vi "Change Color.vi"(8 "error in (no error)":errorcluster, 10 "Color Box":u32, 11 "GObject in":refnum<vi>) -> (0 "error out":errorcluster)   [LabVIEW 2013]
uses:
  Controls/Security System Indicators.ctl
panel:
  out "Zone status indicators":T1
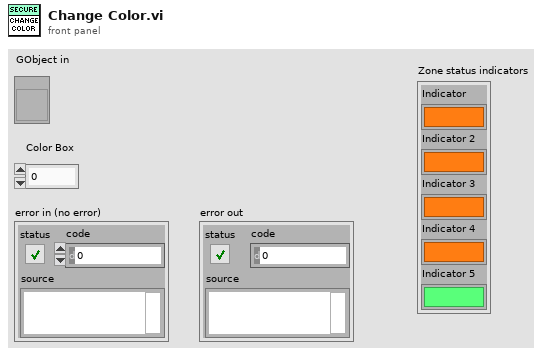
[diagram p1: front panel]
types:
  T1 = typedef "Security System Indicators.ctl" = cluster{"Indicator":bool, "Indicator 2":bool, "Indicator 3":bool, "Indicator 4":bool, "Indicator 5":bool}
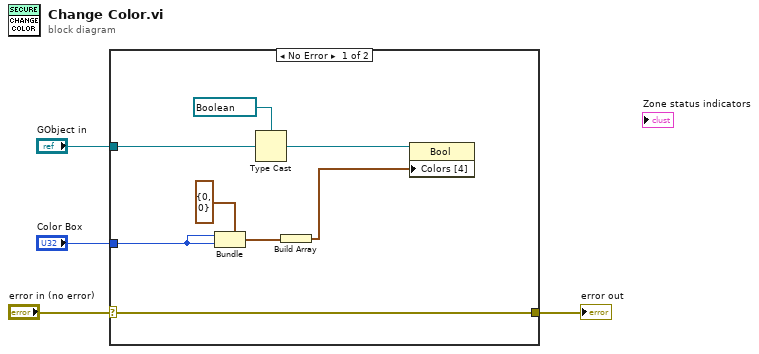
[diagram p0: block diagram]
diagram:
  n1 = case shown="No Error" "error in (no error)" {
    selector: "error in (no error)" -> [w10 w13]
    tunnel: "GObject in" -> [w12 _]
    tunnel: "Color Box" -> [w11 _]
    tunnel: [w10 w13] -> w4
    frame No Error {
      n2 = Bundle(cluster=cluster{"Color Box 2":u32, "Color Box 2":u32} {"Color Box 2"=0, "Color Box 2"=0}, "Color Box 2"=w11, "Color Box 2"=w11) -> (w7:cluster{"Color Box 2":u32, "Color Box 2":u32})
      n3 = Type Cast(type=refnum<vi> refnum ("reference"), x=w12) -> (*(type *) &x=w9:refnum<vi>)
      n4 = Build Array(w7) -> (w6:cluster{"Color Box 2":u32, "Color Box 2":u32}[])
      n5 = property on="Property Node" class="Bool"(reference=w9, "Colors [4]"=w6) -> ()  [unwired: 1 in, 2 out]
    }
    frame Error {
    }
  }
  "error out" <- w4
